vi "SetSystemTimeZone.vi"   [LabVIEW 2017, in "GPTiming.lvlib"]
doc: "Sets the (Windows only) system timezone either by name or by UTC offset (polymorphic).\n\nSteen Schmidt\nGPower"
uses:
  GPTiming.lvlib
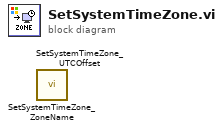
[diagram p0: block diagram]
diagram:
  n1 = call "SetSystemTimeZone_ZoneName.vi"() -> ()  [unwired: 14 in, 2 out]
  n2 = call "SetSystemTimeZone_UTCOffset.vi"() -> ()  [unwired: 14 in, 2 out]
